vi "Convert to Fluofit.vi"() -> ()   [LabVIEW 2009]
uses:
  <vilib>/Utility/file.llb/Read From Spreadsheet File (DBL).vi
panel:
  in  "string to append":string="_all_spots_decays.txt"
  out "output path of created file":path
  in  "All files path":path=path "V:/Tinnefeld/Data/waveguides/20110512 Auswertung/20110427_nochmal/7L/2"
  out "appended array":dbl[][](array[numeric])
  in  "channel of interest":i32=8
  out "all rows":dbl[][](array[numeric]) format="%0.3f"
  # "Merges chosen channel (=row in data file, specified below)\ninto one *.dat file\nChose directiory and all *.dat files are merged for fluofit\nfirst column: time\nall other columns: decays\n\nthe program does this for the specified folder and all\nfollowing folders as long as they are named in increments\ne.g.\n/2\n/3\n/4"
  # "IMPORTANT part : -->"
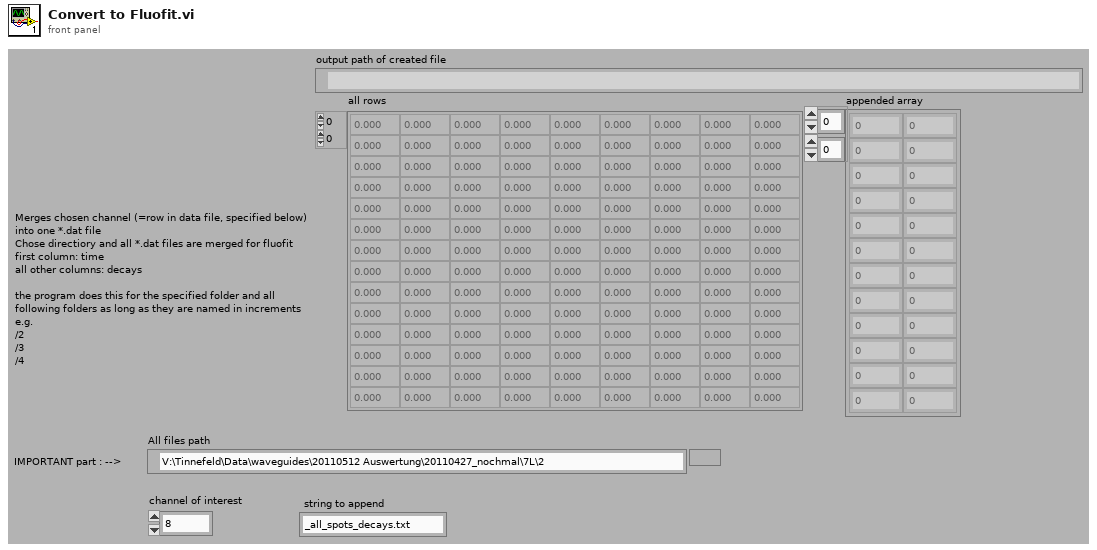
[diagram p1: front panel]
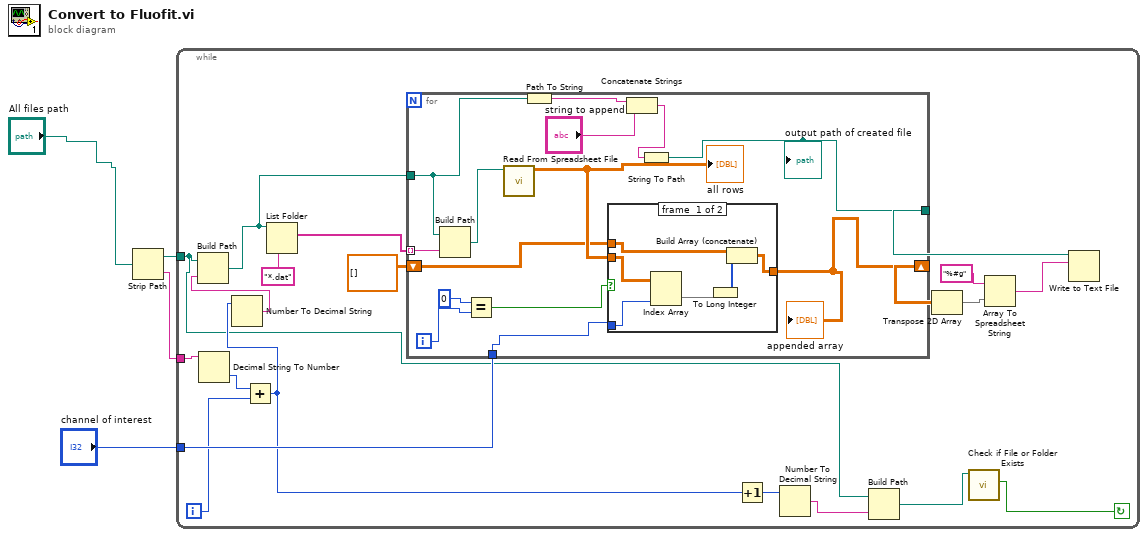
[diagram p0: block diagram]
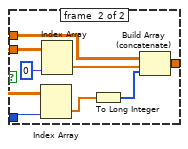
[diagram p2: hidden frame]
diagram:
  n1 = Strip Path(path="All files path") -> (stripped path=w3:path, name=w2:string)
  n2 = while {
    tunnel: "channel of interest" -> [w22]
    tunnel: w3 -> [w5]
    tunnel: w2 -> [w15]
    i -> [w13]
    stop <- w6 continue-if-true
    n3 = Decimal String To Number(string=w15) -> (number=w14:i32)  [unwired: 2 in, 1 out]
    n4 = Add(x=w14, y=w13) -> (x+y=w9:i32)
    n5 = Number To Decimal String(number=w9) -> (decimal integer string=w12:string)  [unwired: 1 in]
    n6 = Build Path(base path=w5, name or relative path=w12) -> (appended path=w11:path)
    n7 = List Folder(path=w11, pattern="*.dat") -> (filenames=w23:string[])  [unwired: 1 in, 4 out]
    n8 = for {
      tunnel: w23 -> [w37] mode=indexing
      tunnel: w22 -> [w36]
      tunnel: w11 -> [w26]
      tunnel: [w32] -> w21
      shift-right: [w30] -> w19
      shift-left: dbl[][] [] -> [w31]
      i -> [w29]
      n9 = Build Path(base path=w26, name or relative path=w37) -> (appended path=w35:path)
      n10 = Equal?(x=0, y=w29) -> (x = y?=w27:bool)
      n11 = call-poly <vilib>:"Read From Spreadsheet File.vi"("file path (dialog if empty)"=w35) -> ("all rows"=w38:dbl[][])  [unwired: 6 in, 4 out]
      "all rows" <- w38
      n12 = Path To String(path=w26) -> (string=w33:string)
      n13 = case shown="False" w27 {
        tunnel: w38 -> [w43 w51]
        tunnel: w36 -> [w44 w49]
        tunnel: w31 -> [w40 w48]
        tunnel: [w41 w47] -> w30
        frame #0 {
          n14 = Index Array(array=w43, index (col)=w44) -> (element=w42:dbl[])  [unwired: 1 in]
          n15 = To Long Integer(number=w42) -> (32bit integer=w39:i32[])
          n16 = Build Array (concatenate)(w40, w39) -> (w41:dbl[][])
        }
        frame #1 {
          n17 = Index Array(array=w51, index (col)=w49) -> (element=w46:dbl[])  [unwired: 1 in]
          n18 = Index Array(array=w51, index (col)=0 ("disabled index (col)")) -> (element=w52:dbl[])  [unwired: 1 in]
          n19 = To Long Integer(number=w46) -> (32bit integer=w45:i32[])
          n20 = Build Array (concatenate)(w48, w52, w45) -> (w47:dbl[][])
        }
      }
      "appended array" <- w30
      n21 = Concatenate Strings(w33, "string to append") -> (w34:string)
      n22 = String To Path(string=w34) -> (path=w32:path)
      "output path of created file" <- w32
    }
    n23 = Increment(x=w9) -> (x+1=w10:i32)
    n24 = Number To Decimal String(number=w10) -> (decimal integer string=w8:string)  [unwired: 1 in]
    n25 = Build Path(base path=w5, name or relative path=w8) -> (appended path=w7:path)
    n26 = Transpose 2D Array(2D array=w19) -> (transposed array=w17:dbl[][])
    n27 = call <vilib>:"Check if File or Folder Exists.vi"("path"=w7) -> ("file or folder exists?"=w6:bool)  [unwired: 8 in, 2 out]
    n28 = Array To Spreadsheet String(array=w17, 3:"%#g" ("format string")) -> (spreadsheet string=w16:string)  [unwired: 1 in]
    n29 = Write to Text File(file (use dialog)=w21, text=w16) -> ()  [unwired: 2 in, 3 out]
  }
